vi "系统交互.vi"   [LabVIEW 2016]
uses:
  PLC/PLC.lvlib
  <vilib>/Utility/config.llb/NI_LVConfig.lvlib
types:
  T1 = typedef "系统交互.ctl" = cluster{"运行模式":enum16{"维护模式", "常规模式", "应急模式", "质控模式"}, "运行间隔":i16, "流程运行中":bool, "自动运行启动参数":cluster{"氨氮":bool, "总磷总氮":bool, "总氮":bool, "CODmn":bool, "CODCr":bool, "超标留样":bool, "多参数":bool}, "SYSTEM Interface.总磷总氮类型":enum16{"单模块", "总磷总氮二合一模块", "氨氮总磷二合一模块"}, "多参数运行间隔":i16}
  T2 = typedef "NI_LVConfig.lvlib/Config Data RefNum.ctl" = refnum<k1>
  T3 = cluster{"氨氮":bool, "总磷总氮":bool, "总氮":bool, "多参数":bool, "CODmn":bool, "CODCr":bool, "超标留样":bool}
  T4 = typedef "模块配置类型.ctl" = enum16{"单模块", "总磷总氮二合一模块", "氨氮总磷二合一模块"}
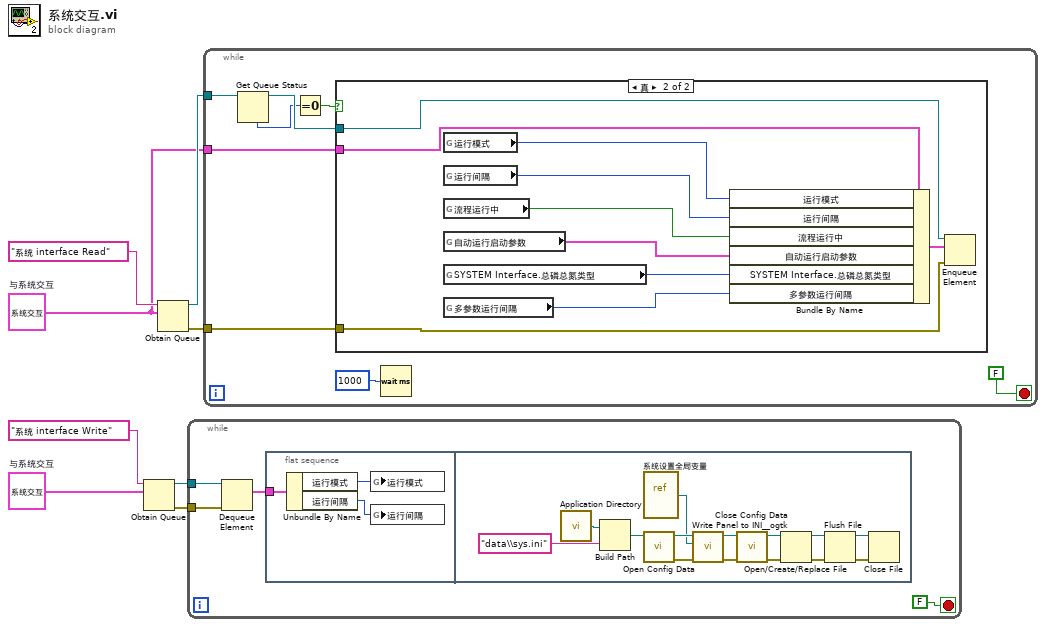
[diagram p0: block diagram]
diagram:
  w4 = T1 {"运行模式"=enum."维护模式", "运行间隔"=4, "流程运行中"=FALSE, "自动运行启动参数"={"氨氮"=FALSE, "总磷总氮"=FALSE, "总氮"=FALSE, "CODmn"=FALSE, "CODCr"=FALSE, "超标留样"=FALSE, "多参数"=FALSE}, "SYSTEM Interface.总磷总氮类型"=enum."单模块", "多参数运行间隔"=4}  # 与系统交互
  w5 = T1 {"运行模式"=enum."维护模式", "运行间隔"=4, "流程运行中"=FALSE, "自动运行启动参数"={"氨氮"=FALSE, "总磷总氮"=FALSE, "总氮"=FALSE, "CODmn"=FALSE, "CODCr"=FALSE, "超标留样"=FALSE, "多参数"=FALSE}, "SYSTEM Interface.总磷总氮类型"=enum."单模块", "多参数运行间隔"=4}  # 与系统交互
  n1 = Obtain Queue(name (unnamed)="系统 interface Write" ("写入方名称"), element data type=w4) -> (queue out=w2:refnum<queue>, error out=w3:errorcluster)  [unwired: 3 in, 1 out]
  n2 = Obtain Queue(name (unnamed)="系统 interface Read" ("写入方名称"), element data type=w5) -> (queue out=w7:refnum<queue>, error out=w6:errorcluster)  [unwired: 3 in, 1 out]
  n3 = while {
    tunnel: w2 -> [w11]
    tunnel: w3 -> [w10]
    stop <- FALSE stop-if-true
    n4 = Dequeue Element(queue=w11, error in (no error)=w10) -> (element=w9:T1)  [unwired: 1 in, 3 out]
    n5 = flat-sequence {
      tunnel: w9 -> [w13]
      frame #0 {
        n6 = Unbundle By Name(w13) -> ("运行模式"=w14:enum16{"维护模式", "常规模式", "应急模式", "质控模式"}, "运行间隔"=w15:i16)
        n7 = global write "系统设置全局变量.vi" "运行模式"(w14) -> ()
        n8 = global write "系统设置全局变量.vi" "运行间隔"(w15) -> ()
      }
      frame #1 {
        n9 = call <vilib>:"Application Directory.vi"() -> ("Application Directory"=w29:path)
        n10 = Build Path(base path=w29, name or relative path="data\\sys.ini" ("名称或相对路径")) -> (appended path=w27:path)
        n11 = vi-ref "系统设置全局变量.vi"() -> (w25:refnum<vi>)
        n12 = call <vilib>:"Open Config Data.vi"("configuration file path"=w27) -> ("error out"=w23:errorcluster, "refnum"=w26:T2)  [unwired: 8 in, 1 out]
        n13 = call <userlib>:"Write Panel to INI__ogtk.vi"("error in (no error)"=w23, "VI ref"=w25, "refnum"=w26) -> ("error out"=w22:errorcluster, "refnum out"=w24:T2)  [unwired: 7 in]
        n14 = call <vilib>:"Close Config Data.vi"("error in (no error)"=w22, "refnum"=w24) -> ("error out"=w17:errorcluster, "file path"=w16:path)  [unwired: 8 in]
        n15 = Open/Create/Replace File(file path (use dialog)=w16, error in=w17) -> (refnum out=w20:refnum<file>, error out=w21:errorcluster)  [unwired: 4 in, 1 out]
        n16 = Flush File(refnum=w20, error in=w21) -> (refnum out=w19:refnum<file>, error out=w18:errorcluster)
        n17 = Close File(refnum=w19, error in=w18) -> ()  [unwired: 2 out]
      }
    }
  }
  n18 = while {
    tunnel: w7 -> [w35]
    tunnel: w6 -> [w34]
    tunnel: w5 -> [w33]
    stop <- FALSE stop-if-true
    n19 = Get Queue Status(queue=w35) -> (queue out=w32:refnum<queue>, # elements in queue=w31:i32)  [unwired: 2 in, 6 out]
    n20 = Equal To 0?(x=w31) -> (x = 0?=w30:bool)
    n21 = case shown="真" w30 {
      tunnel: w34 -> [_ w47]
      tunnel: w33 -> [_ w46]
      tunnel: w32 -> [_ w40]
      frame False {
      }
      frame True {
        n22 = global read "系统设置全局变量.vi" "运行模式"() -> (w45:enum16{"维护模式", "常规模式", "应急模式", "质控模式"})
        n23 = global read "系统设置全局变量.vi" "运行间隔"() -> (w44:i16)
        n24 = global read "采配水全局变量.vi" "流程运行中"() -> (w43:bool)
        n25 = global read "系统设置全局变量.vi" "自动运行启动参数"() -> (w42:T3)
        n26 = global read "系统设置全局变量.vi" "SYSTEM Interface.总磷总氮类型"() -> (w38:T4)
        n27 = global read "系统设置全局变量.vi" "多参数运行间隔"() -> (w39:i16)
        n28 = Bundle By Name(cluster=w46, "运行模式"=w45, "运行间隔"=w44, "流程运行中"=w43, "自动运行启动参数"=w42, "SYSTEM Interface.总磷总氮类型"=w38, "多参数运行间隔"=w39) -> (w41:T1)
        n29 = Enqueue Element(queue=w40, element=w41, error in (no error)=w47) -> ()  [unwired: 1 in, 3 out]
      }
    }
    n30 = Wait (ms)(milliseconds to wait=u32 1000 ("等待时间（毫秒）")) -> ()  [unwired: 1 out]
  }
